vi "Build Array.vi"() -> ()   [LabVIEW 2019]
panel:
  in  "?":bool
  out "Output Array":dbl[](array[numeric])
  in  "Index":i32
  in  "Element to insert":dbl
  in  "?":bool
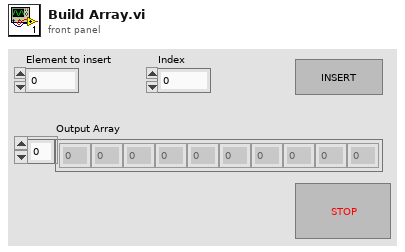
[diagram p1: front panel]
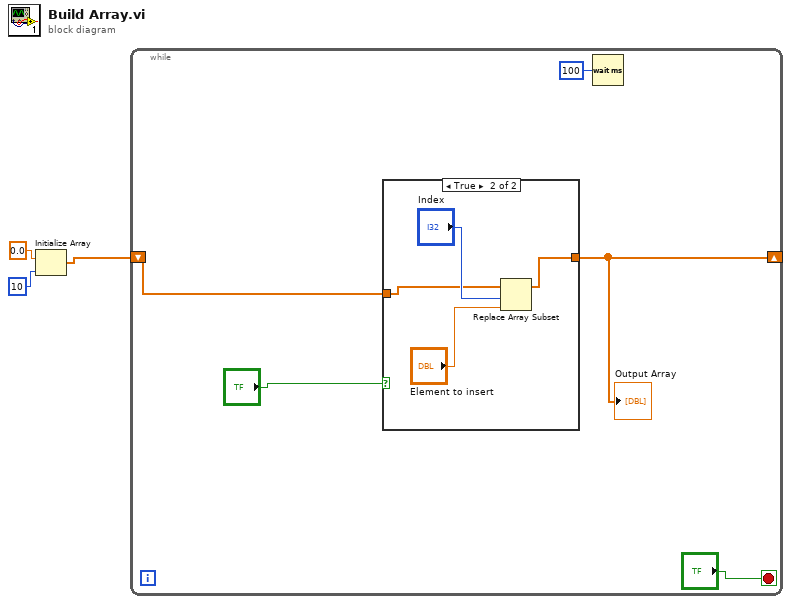
[diagram p0: block diagram]
diagram:
  n1 = Initialize Array(0.0 ("element"), 10 ("dimension size")) -> (w1:dbl[])
  n2 = while {
    shift-right: [w4] -> _
    shift-left: w1 -> [w6]
    stop <- "?" stop-if-true
    n3 = case shown="True" "?" {
      tunnel: w6 -> [w9 w10]
      tunnel: [w9 w11] -> w4
      frame False {
      }
      frame True {
        n4 = Replace Array Subset(array=w10, new element="Element to insert", index="Index") -> (w11:dbl[])
      }
    }
    "Output Array" <- w4
    n5 = Wait (ms)(milliseconds to wait=u32 100) -> ()  [unwired: 1 out]
  }
